vi "ReadVoltage.vi"(8 "Error In":errorcluster, 11 "reference in":refnum<class "VdAnalogInput_Simulated.lvclass">) -> (0 "Error Out":errorcluster, 2 "Voltage":dbl, 3 "reference in":refnum<class "VdAnalogInput_Simulated.lvclass">)   [LabVIEW 2020, in "VdAnalogInput_Simulated.lvclass"]
uses:
  VdAnalogInput_Simulated.lvclass
  VdAnalogInput_Simulated.lvclass/VdAnalogInput_Simulated.ctl
  VdAnalogInput_class/VdAnalogInput.lvclass
  <vilib>/numeric/Random Number (Range) DBL.vi
  C:/Projects/DesignPatterns/Factory1/VdAnalogInput_class/VdAnalogInput.lvclass
  C:/Projects/DesignPatterns/Factory1/VdInstrument_class/VdInstrument.lvclass
  C:/Projects/DesignPatterns/Factory1/VdAnalogInput_Simulated_class/VdAnalogInput_Simulated.lvclass
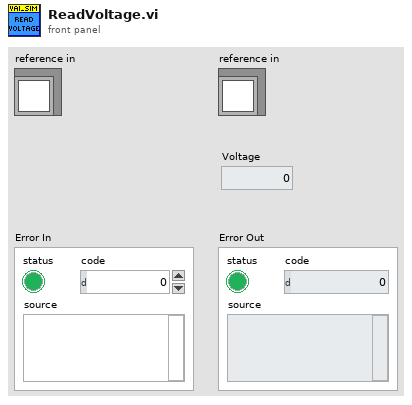
[diagram p1: front panel]
types:
  T1 = typedef "VdAnalogInput.lvclass/ObjectAttributes.ctl" = cluster{"LastReadValue":dbl, "VoltageRangeLow":dbl, "VoltageRangeHigh":dbl}
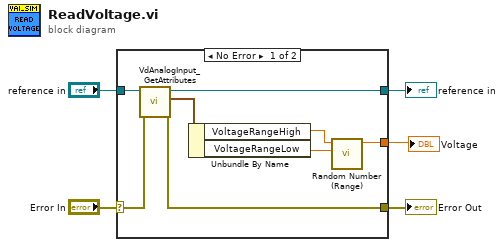
[diagram p0: block diagram]
diagram:
  n1 = case shown="No Error" "Error In" {
    selector: "Error In" -> [w13 w15]
    tunnel: [w11 w15] -> w4
    tunnel: [w9 w14] -> w2
    tunnel: "reference in" -> [w10 w14]
    tunnel: [w6 _] -> w1
    frame No Error {
      n2 = call "VdAnalogInput_GetAttributes.vi"("error in (no error)"=w13, "reference in"=w10) -> ("error out"=w11:errorcluster, "Data"=w12:T1, "reference out"=w9:refnum<class "VdAnalogInput_Simulated.lvclass">)  [unwired: 6 in, 1 out]
      n3 = Unbundle By Name(w12) -> ("VoltageRangeHigh"=w8:dbl, "VoltageRangeLow"=w7:dbl)
      n4 = call-poly <vilib>:"Random Number (Range).vi"("lower bound (0)"=w7, "upper bound (100)"=w8) -> ("number"=w6:dbl)  [unwired: 9 in]
    }
    frame Error {
    }
  }
  "Error Out" <- w4
  "reference in" <- w2
  "Voltage" <- w1
